vi "Project 2016.vi"() -> ()   [LabVIEW 2016]
uses:
  <vilib>/MakerHub/LINX/LMH-LINX.lvlib
  <vilib>/MakerHub/LINX/Public/Peripherals/Analog/Analog Read 1 Chan.vi
  <vilib>/MakerHub/LINX/Public/Utilities/Open Serial.vi
  <vilib>/MakerHub/LINX/Public/Peripherals/Digital/Digital Write 1 Chan.vi
panel:
  out "Smoke":dbl(graph)
  out "SMOKE":dbl
  out "Thermometer":dbl(slide) scale=20.0..40.0
  out "Temperature":dbl
  in  "stop":bool
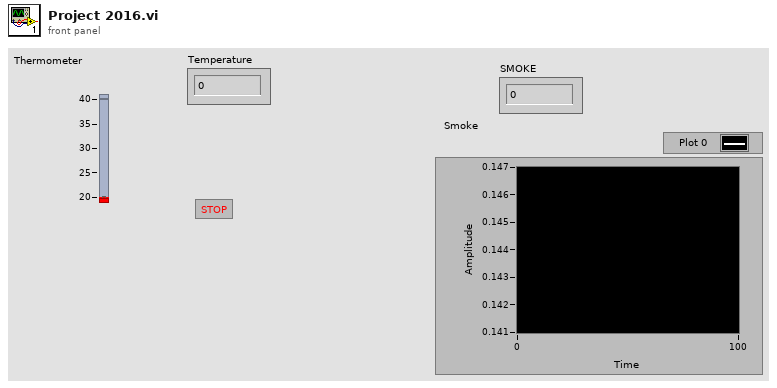
[diagram p1: front panel]
types:
  T1 = typedef "LMH-LINX.lvlib/LINX Ref.ctl" = cluster{"IO":T2, "Interface":T3, "LINX Device Config":T4}
  T2 = typedef "LMH-LINX.lvlib/Platform.ctl" = enum16{"Remote", "Local"}
  T3 = typedef "LMH-LINX.lvlib/Interface.ctl" = enum16{"Serial", "TCP"}
  T4 = typedef "LMH-LINX.lvlib/Device.lvlib/LINX Device Config.ctl" = cluster{"Interface":T3, "COM Port":refnum<visa-resource-name>, "TCP Configuration":T5, "Device Family":u8, "Device ID":u8, "Device Name":string, "TCP Ref":refnum<k5>, "Channels":T6}
  T5 = typedef "LMH-LINX.lvlib/Device.lvlib/TCP Config.ctl" = cluster{"IP Address":string, "Port":u16}
  T6 = typedef "LMH-LINX.lvlib/Channels.ctl" = cluster{"DI":u8[], "DO":u8[], "AI":u8[], "AO":u8[], "PWM":u8[], "QE":u8[], "UART":u8[], "I2C 2":u8[], "SPI":u8[], "CAN":u8[], "Servo":u8[], "AI Ref (V)":dbl, "AI Resolution (Bits)":u8, "AO Ref (V)":dbl, "AO Resolution (Bits)":u8}
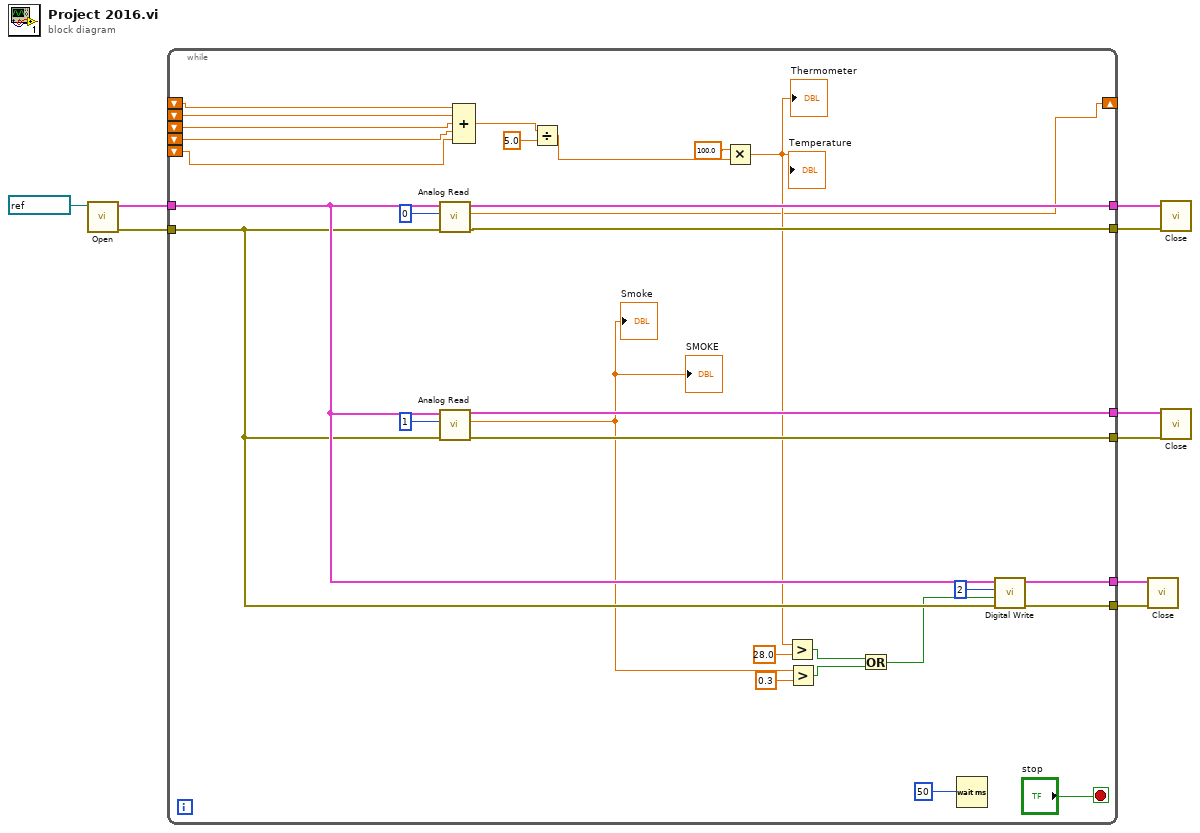
[diagram p0: block diagram]
diagram:
  n1 = call-poly <vilib>:"Open.vi"("Serial Port"=refnum<visa-resource-name> "COM9") -> ("Error Out"=w6:errorcluster, "LINX Resource"=w9:T1)  [unwired: 8 in, 1 out]
  n2 = while {
    tunnel: w9 -> [w30]
    tunnel: [w37] -> w8
    tunnel: [w36] -> w7
    tunnel: w6 -> [w29]
    tunnel: [w33] -> w4
    tunnel: [w32] -> w3
    tunnel: [w28] -> w2
    tunnel: [w27] -> w1
    shift-right: [w18] -> _
    shift-left: _ -> [w17]
    shift-left: _ -> [w16]
    shift-left: _ -> [w15]
    shift-left: _ -> [w14]
    shift-left: _ -> [w13]
    stop <- "stop" stop-if-true
    n3 = call-poly <vilib>:"Analog Read.vi"("Error In"=w29, "Analog Channel"=u8 0, "LINX Resource"=w30) -> ("Error Out"=w36:errorcluster, "Voltage"=w18:dbl, "LINX Resource"=w37:T1)  [unwired: 5 in, 1 out]
    n4 = call-poly <vilib>:"Analog Read.vi"("Error In"=w29, "Analog Channel"=u8 1, "LINX Resource"=w30) -> ("Error Out"=w32:errorcluster, "Voltage"=w20:dbl, "LINX Resource"=w33:T1)  [unwired: 5 in, 1 out]
    "SMOKE" <- w20
    "Smoke" <- w20
    n5 = Compound Arithmetic op=ADD(w17, w16, w15, w14, w13) -> (w10:dbl)
    n6 = Divide(x=w10, y=5.0) -> (x/y=w11:dbl)
    n7 = Multiply(x=100.0, y=w11) -> (x*y=w19:dbl)
    "Temperature" <- w19
    "Thermometer" <- w19
    n8 = Greater?(x=w19, y=28.0) -> (0:w24:bool)
    n9 = Greater?(x=w20, y=0.3) -> (0:w23:bool)
    n10 = Or(x=w24, y=w23) -> (x .or. y?=w25:bool)
    n11 = Wait (ms)(milliseconds to wait=u32 50 ("millisecond timer value")) -> ()  [unwired: 1 out]
    n12 = call-poly <vilib>:"Digital Write.vi"("Error In"=w29, "Output Value"=w25, "DO Channel"=u8 2, "LINX Resource"=w30) -> ("Error Out"=w27:errorcluster, "LINX Resource"=w28:T1)  [unwired: 6 in]
  }
  n13 = call <vilib>:"Close.vi"("Error In"=w1, "LINX Resource"=w2) -> ()  [unwired: 9 in, 1 out]
  n14 = call <vilib>:"Close.vi"("Error In"=w7, "LINX Resource"=w8) -> ()  [unwired: 9 in, 1 out]
  n15 = call <vilib>:"Close.vi"("Error In"=w3, "LINX Resource"=w4) -> ()  [unwired: 9 in, 1 out]
